vi "Invalid CLI parameter input--error.vi"() -> (0 "error out":errorcluster)   [LabVIEW 2025]
doc: "Indicates that the specified CLI command/parameter combination is invalid (e.g. user typed launch but no --name)."
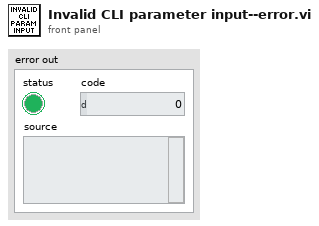
[diagram p1: front panel]
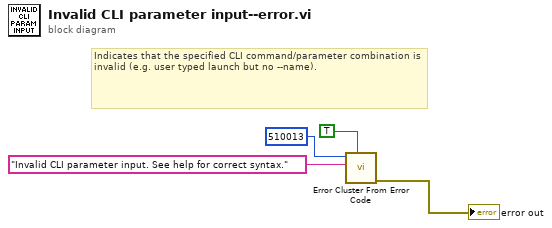
[diagram p0: block diagram]
diagram:
  # "Indicates that the specified CLI command/parameter combination is invalid (e.g. user typed launch but no --name)."
  n1 = call <vilib>:"Error Cluster From Error Code.vi"("show call chain? (False)"=TRUE, "error message (\"\")"="Invalid CLI parameter input. See help for correct syntax." ("error message (\"\")"), "error code (0)"=510013) -> ("error out"=→"error out":errorcluster)  [unwired: 6 in]
